vi "solar_voy Destroy.vi"(6 "Suppress Errors? (T)":bool=TRUE, 8 "error in (no error)":errorcluster, 11 "Voyager Refnum":T1) -> (0 "error out":errorcluster)   [LabVIEW 2018]
doc: "This destroys the Voyager reference and closes all TCP ports."
uses:
  solar_voy_ctl Voyager Refnum.ctl
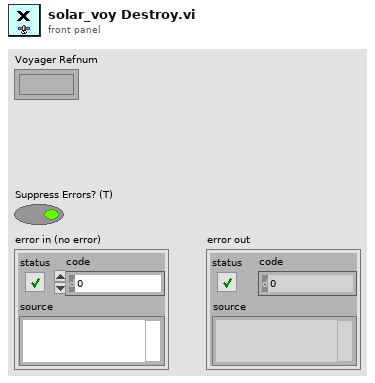
[diagram p1: front panel]
types:
  T1 = typedef "solar_voy_ctl Voyager Refnum.ctl" = refnum<k1>
  T2 = typedef "solar_voy_ctl Voyager.ctl" = cluster{"PACKETS":T3[], "COSMOS_Root":path, "CMD_HDR":T8, "TLM_HDR":T8, "TCPs":T9[], "VoyagerIDOffset":cluster{"VoyagerIDOffset":u16[], "Target Names":string[]}}
  T3 = typedef "solar_voy_def_ctl PACKET.ctl" = cluster{"PACKET_ID":T4, "ENDIAN":enum8{"BIG", "LITTLE"}, "DESC":string, "HZRD":bool, "ITEMS":T5[], "NoExport":bool, "last_time":timestamp, "last_count":u32, "last_data":string}
  T4 = typedef "solar_voy_def_ctl PACKET_ID.ctl" = cluster{"ID":u16, "CMD":enum8{"CMD", "TLM"}, "TARGET":string, "PACKET":string}
  T5 = typedef "solar_voy_def_ctl ITEM.ctl" = cluster{"NAME":string, "OFFSET":i32, "SIZE":i32, "TYPE":T6, "EACH_SIZE":i32, "LVTYPE":T7, "MIN":dbl, "MAX":dbl, "DEFAULT":string, "DESC":string, "ID":bool, "MODIFIERS":variant, "last_value":variant}
  T6 = typedef "solar_voy_def_ctl ITEM TYPE.ctl" = enum8{"BLOCK", "INT", "UINT", "FLOAT", "STRING"}
  T7 = typedef "solar_type Item Type.ctl" = enum16{"NULL", "UNKNOWN", "CLUSTER", "I8", "I16", "I32", "I64", "U8", "U16", "U32", "U64", "U8_ENUM", "U16_ENUM", "U32_ENUM", "SGL", "DBL", "BOOLEAN", "STRING", "PATH", "VISA", "TAG", "TIME", "I8_1D", "I16_1D", "I32_1D", "I64_1D", "U8_1D", "U16_1D", "U32_1D", "U64_1D", "U8_ENUM_1D", "U16_ENUM_1D", "U32_ENUM_1D", "SGL_1D", "DBL_1D", "BOOLEAN_1D", "STRING_1D", "PATH_1D", "VISA_1D", "TAG_1D", "TIME_1D", "I8_2D", "I16_2D", "I32_2D", "I64_2D", "U8_2D", "U16_2D", "U32_2D", "U64_2D", "U8_ENUM_2D", "U16_ENUM_2D", "U32_ENUM_2D", "SGL_2D", "DBL_2D", "BOOLEAN_2D", "STRING_2D", "PATH_2D", "VISA_2D", "TAG_2D", "TIME_2D"}
  T8 = typedef "solar_voy_def_ctl HDR.ctl" = cluster{"ITEMS":T5[], "LENGTH_NAME":string, "LENGTH_VALUE_OFFSET":i32, "ID_NAME":string, "ENDIAN":enum8{"BIG", "LITTLE"}, "GUID_NAME":string, "DEFAULT_TARGET":string, "DEFAULT_PACKET":string, "DEFAULT_ERROR":string}
  T9 = typedef "solar_voy_ctl TCP.ctl" = cluster{"Connected":bool, "Port":u16, "Listener":refnum<k5>, "ServerIP":string, "TCP":refnum<k5>, "Setup":T10, "VIRefnum":refnum<vi>, "TARGETS_CMD":string[], "TARGETS_TLM":string[]}
  T10 = typedef "solar_voy_ctl Port Setup.ctl" = enum8{"SERVER", "CLIENT", "SERVER_CMD", "SERVER_TLM"}
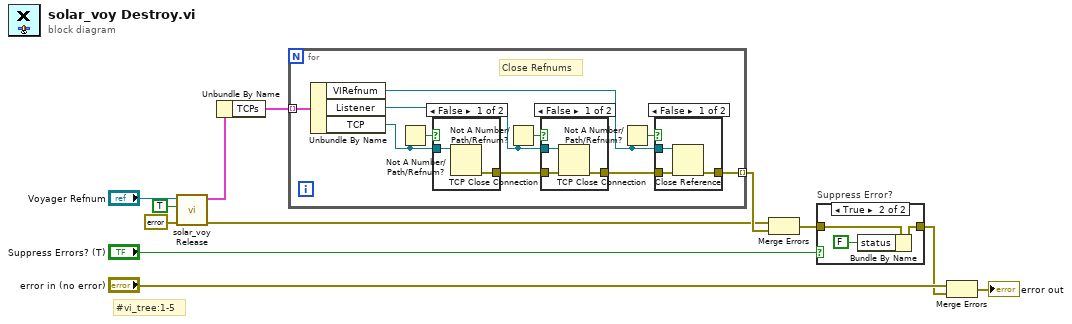
[diagram p0: block diagram]
diagram:
  # "#vi_tree:1-5"
  n1 = call "solar_voy Release.vi"("error in (no error)"=errorcluster {"status"=FALSE, "code"=0, "source"=""}, "Force Destroy? (F)"=TRUE, "Voyager Refnum"="Voyager Refnum") -> ("error out"=w1:errorcluster, "Voyager"=w5:T2)  [unwired: 7 in]
  n2 = Unbundle By Name(w5) -> ("TCPs"=w4:T9[])
  n3 = for {
    tunnel: w4 -> [w22] mode=indexing
    tunnel: [w13] -> w3 mode=indexing
    # "Close Refnums"
    n4 = Unbundle By Name(w22) -> ("VIRefnum"=w14:refnum<vi>, "Listener"=w17:refnum<k5>, "TCP"=w21:refnum<k5>)
    n5 = Not A Number/Path/Refnum?(number/path/refnum=w21) -> (NaN/Path/Refnum?=w20:bool)
    n6 = case shown="False" w20 {
      tunnel: [w32 _] -> w18
      tunnel: w21 -> [w31 _]
      frame False {
        n7 = TCP Close Connection(connection ID=w31) -> (error out=w32:errorcluster)  [unwired: 2 in, 1 out]
      }
      frame True {
      }
    }
    n8 = Not A Number/Path/Refnum?(number/path/refnum=w17) -> (NaN/Path/Refnum?=w19:bool)
    n9 = case shown="False" w19 {
      tunnel: w18 -> [w29 w30]
      tunnel: [w28 w30] -> w15
      tunnel: w17 -> [w27 _]
      frame False {
        n10 = TCP Close Connection(connection ID=w27, error in (no error)=w29) -> (error out=w28:errorcluster)  [unwired: 1 in, 1 out]
      }
      frame True {
      }
    }
    n11 = Not A Number/Path/Refnum?(number/path/refnum=w14) -> (NaN/Path/Refnum?=w16:bool)
    n12 = case shown="False" w16 {
      tunnel: w15 -> [w25 w26]
      tunnel: [w24 w26] -> w13
      tunnel: w14 -> [w23 _]
      frame False {
        n13 = Close Reference(reference=w23, error in (no error)=w25) -> (error out=w24:errorcluster)
      }
      frame True {
      }
    }
  }
  n14 = Merge Errors(w1, w3) -> (w2:errorcluster)
  n15 = case "Suppress Error?" shown="True" "Suppress Errors? (T)" {
    tunnel: w2 -> [w33 w36]
    tunnel: [w33 w35] -> w10
    frame False {
    }
    frame True {
      n16 = Bundle By Name(cluster=w36, "status"=FALSE) -> (w35:errorcluster)
    }
  }
  n17 = Merge Errors("error in (no error)", w10) -> (→"error out":errorcluster)
